vi "OD Factor.vi"(1 "LNAttenuation":dbl, 2 "Linewidth":dbl[unit]=5234000.0, 3 "Detuning":dbl[unit]=10000000.0) -> (0 "Optical Density":dbl)   [LabVIEW 2009]
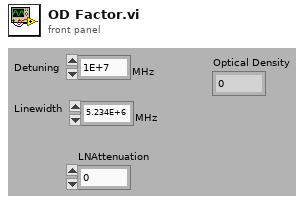
[diagram p1: front panel]
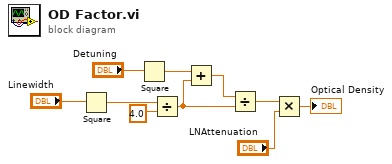
[diagram p0: block diagram]
diagram:
  n1 = Square(x="Linewidth") -> (x^2=w2:dbl[unit])
  n2 = Square(x="Detuning") -> (x^2=w4:dbl[unit])
  n3 = Divide(x=w2, y=4.0) -> (x/y=w7:dbl[unit])
  n4 = Add(x=w4, y=w7) -> (x+y=w6:dbl[unit])
  n5 = Divide(x=w6, y=w7) -> (x/y=w9:dbl)
  n6 = Multiply(x=w9, y="LNAttenuation") -> (x*y=→"Optical Density":dbl)
